vi "FPGAcode4.vi"() -> ()   [LabVIEW 2015]
uses:
  Limits_In.ctl
  Detector_Cluster.ctl
  <vilib>/Platform/TimedLoop/XDataNode/timing_clust.ctl
  <vilib>/Platform/TimedLoop/XDataNode/nitl_modes.ctl
  <vilib>/Platform/TimedLoop/XDataNode/wakeup.ctl
  Correlations.ctl
  <vilib>/rvi/Emulation/niFpgaSctlEmulationGetInTimedLoop.vi
  <vilib>/rvi/Emulation/niFpgaEmulationReportErrorSimple.vi
  <vilib>/rvi/Emulation/niFpgaGetClockAttributes.vi
  <vilib>/rvi/Emulation/niFpgaCriticalErrorInLSC.vi
  <vilib>/rvi/eio/common/nirviEmuTemplateMethod_errors.vi
  <vilib>/rvi/Emulation/niFpgaEmulationIsFPGAContextNoSignature.vi
  <vilib>/rvi/DataTransferAndStorage/Container/Common/niFpgaContainerGetUniqueNameForEmu.vi
  <vilib>/rvi/eio/common/nirviEmuReportErrorAndStop.vi
  <vilib>/rvi/Emulation/niFpgaProcessEmulError.vi
  <vilib>/Platform/TimedLoop/XDataNode/XDataNode.xnode
  <vilib>/eio/EIONode/EIONode.xnode
  <vilib>/rvi/DataTransferAndStorage/Container/XNode/niFpgaContainer.xnode
  <vilib>/rvi/DataTransferAndStorage/Handshake/Emulation/niFpgaHandshakeEmulation.vi
  <vilib>/Platform/TimedLoop/XDataNode/XDNodeRunTimeDep.lvlib
panel:
  in  "Charge Error Factor":fxp<+/-,11,1>=0.2001953125 format="%#.3g"
  in  "Calibrate":bool=TRUE
  in  "Limits":T1={"High Charge Limit"=4.54747350780585e-13, "Low Charge Limit"=0.0, "High Velocity Limit"=262143.0, "Low Velocity Limit"=0.0, "High Mass Limit"=7.27595761248936e-12, "Low Mass Limit"=0.0, "High Voltage"=2200000.0}
  in  "One Shot":bool
  in  "Threshold Factor":fxp<+,12,2>=1.150390625 format="%#.3g"
  in  "Armed":bool
  in  "User Trigger Distance":fxp<+/-,28,18> format="%#.3g"
  in  "User Trigger?":bool
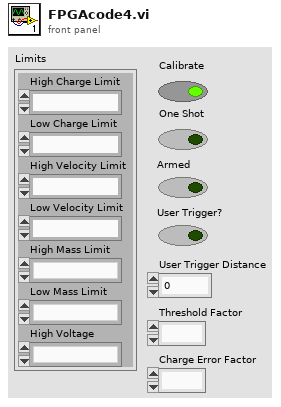
[diagram p1: front panel]
types:
  T1 = typedef "Limits_In.ctl" = cluster{"High Charge Limit":fxp<+,32,-41>, "Low Charge Limit":fxp<+,32,-41>, "High Velocity Limit":fxp<+,18,18>, "Low Velocity Limit":fxp<+,18,18>, "High Mass Limit":fxp<+,32,-37>, "Low Mass Limit":fxp<+,32,-37>, "High Voltage":fxp<+,22,22>}
  T2 = cluster{"[0]":fxp<+,16,1>, "[1]":fxp<+,16,1>, "[2]":fxp<+,16,1>, "[3]":fxp<+,16,1>, "[4]":fxp<+,16,1>, "[5]":fxp<+,16,1>, "[6]":fxp<+,16,1>, "[7]":fxp<+,16,1>, "[8]":fxp<+,16,1>, "[9]":fxp<+,16,1>, "[10]":fxp<+,16,1>}
  T3 = cluster{"[0]":i32, "[1]":i32, "[2]":i32, "[3]":i32, "[4]":i32, "[5]":i32, "[6]":i32, "[7]":i32, "[8]":i32, "[9]":i32, "[10]":i32}
  T4 = cluster{"[0]":cluster{"Detector Max Speed Count":i32, "Detector Min Speed Count":i32, "Gap Max Speed Count":i32, "Gap Min Speed Count":i32}, "[1]":cluster{"Detector Max Speed Count":i32, "Detector Min Speed Count":i32, "Gap Max Speed Count":i32, "Gap Min Speed Count":i32}, "[2]":cluster{"Detector Max Speed Count":i32, "Detector Min Speed Count":i32, "Gap Max Speed Count":i32, "Gap Min Speed Count":i32}, "[3]":cluster{"Detector Max Speed Count":i32, "Detector Min Speed Count":i32, "Gap Max Speed Count":i32, "Gap Min Speed Count":i32}, "[4]":cluster{"Detector Max Speed Count":i32, "Detector Min Speed Count":i32, "Gap Max Speed Count":i32, "Gap Min Speed Count":i32}, "[5]":cluster{"Detector Max Speed Count":i32, "Detector Min Speed Count":i32, "Gap Max Speed Count":i32, "Gap Min Speed Count":i32}, "[6]":cluster{"Detector Max Speed Count":i32, "Detector Min Speed Count":i32, "Gap Max Speed Count":i32, "Gap Min Speed Count":i32}, "[7]":cluster{"Detector Max Speed Count":i32, "Detector Min Speed Count":i32, "Gap Max Speed Count":i32, "Gap Min Speed Count":i32}, "[8]":cluster{"Detector Max Speed Count":i32, "Detector Min Speed Count":i32, "Gap Max Speed Count":i32, "Gap Min Speed Count":i32}, "[9]":cluster{"Detector Max Speed Count":i32, "Detector Min Speed Count":i32, "Gap Max Speed Count":i32, "Gap Min Speed Count":i32}, "[10]":cluster{"Detector Max Speed Count":i32, "Detector Min Speed Count":i32, "Gap Max Speed Count":i32, "Gap Min Speed Count":i32}}
  T5 = cluster{cluster{"[0]":i32, "[1]":i32, "[2]":i32, "[3]":i32, "[4]":i32, "[5]":i32, "[6]":i32, "[7]":i32, "[8]":i32, "[9]":i32, "[10]":i32}, cluster{"[0]":i32, "[1]":i32, "[2]":i32, "[3]":i32, "[4]":i32, "[5]":i32, "[6]":i32, "[7]":i32, "[8]":i32, "[9]":i32, "[10]":i32}, cluster{"[0]":i32, "[1]":i32, "[2]":i32, "[3]":i32, "[4]":i32, "[5]":i32, "[6]":i32, "[7]":i32, "[8]":i32, "[9]":i32, "[10]":i32}, cluster{"[0]":i32, "[1]":i32, "[2]":i32, "[3]":i32, "[4]":i32, "[5]":i32, "[6]":i32, "[7]":i32, "[8]":i32, "[9]":i32, "[10]":i32}}
  T6 = cluster{"Distance to PSU":fxp<+/-,64,37>, "Distance to end of PSU":fxp<+/-,64,37>, "Distance to DCS 2":fxp<+/-,64,37>, "Distance to DCS 1":fxp<+/-,64,37>, "Distance to front of LEIL Chamber":fxp<+/-,64,37>}
  T7 = typedef "Detector_Cluster.ctl" = cluster{"Det 1":i32, "Det 2":i32}
  T8 = cluster{"Filter 1":T7, "Filter 2":T7, "Filter 3":T7, "Filter 4":T7}
  T9 = cluster{"Detector Max Speed Count":i32, "Detector Min Speed Count":i32, "Gap Max Speed Count":i32, "Gap Min Speed Count":i32}[]
  T10 = cluster{"Filter 1":T7, "Filter 2":T7, "Filter 3":T7, "Filter 4":T7}[]
  T11 = typedef "XDNodeRunTimeDep.lvlib/timing_clust.ctl" = cluster{"Expected End [f-1]":u64, "Actual End [f-1]":u64, "Finished Late? [f-1]":bool, "Expected End [i-1]":u64, "Actual End [i-1]":u64, "Finished Late? [i-1]":bool, "Expected Start [i]":u64, "Actual Start [i]":u64, "Expected Start [f]":u64, "Actual Start [f]":u64, "Source Name":string, "Structure Name":string, "Period":i64, "Deadline":i64, "Offset":i64, "Start":i64, "Priority":i32, "Timeout":i32, "Mode":T12, "Wakeup Reason":T13, "Error":errorcluster, "Source Type":string, "Secondary Source Type":string, "Global End Time":u64, "Global Start Time":u64, "Frame Duration":u64, "Iteration Duration":u64, "Assigned CPU":i32, "I/O Scan Engine Mode":u32}
  T12 = typedef "XDNodeRunTimeDep.lvlib/nitl_modes.ctl" = enum32{"No Change", "Process missed periods, maintain original phase", "Discard missed periods, maintain original phase", "Process missed periods, ignore original phase", "Discard missed periods, ignore original phase"}
  T13 = typedef "XDNodeRunTimeDep.lvlib/wakeup.ctl" = enum32{"Normal", "Aborted", "Asynchronous wakeup", "Timing source error", "Timed loop error", "Timeout"}
  T14 = cluster{"IO Module\\AI 0":i16, "IO Module\\AI 1":i16}
  T15 = cluster{"First Detector Count":i32, "Detector Gap Count":i32, "Second Detector Count":i32, "Second Detector Final Count":i32}
  T16 = typedef "Correlations.ctl" = cluster{"First Correlation":i32, "Latest Correlation":i32}
  T17 = cluster{"Data":fxp<+/-,40,32>, "Data":fxp<+/-,40,32>}
  T18 = cluster{cluster{"Data":i16, "Data":i16}, cluster{"Det 1":i16, "Det 2":i16}, cluster{"Det 1":i16, "Det 2":i16}, cluster{"Det 1":i16, "Det 2":i16}}
  T19 = cluster{cluster{"Det 1":i16, "Det 2":i16}, cluster{"Det 1":i16, "Det 2":i16}, cluster{"Det 1":i16, "Det 2":i16}, cluster{"Det 1":i16, "Det 2":i16}}
  T20 = cluster{"Distance to PSU":fxp<+/-,64,69>, "Distance to end of PSU":fxp<+/-,64,69>, "Distance to DCS 2":fxp<+/-,64,69>, "Distance to DCS 1":fxp<+/-,64,69>, "Distance to front of LEIL Chamber":fxp<+/-,64,69>}
  T21 = cluster{"Distance to PSU":i32, "Distance to end of PSU":i32, "Distance to DCS 2":i32, "Distance to DCS 1":i32, "Distance to front of LEIL Chamber":i32}
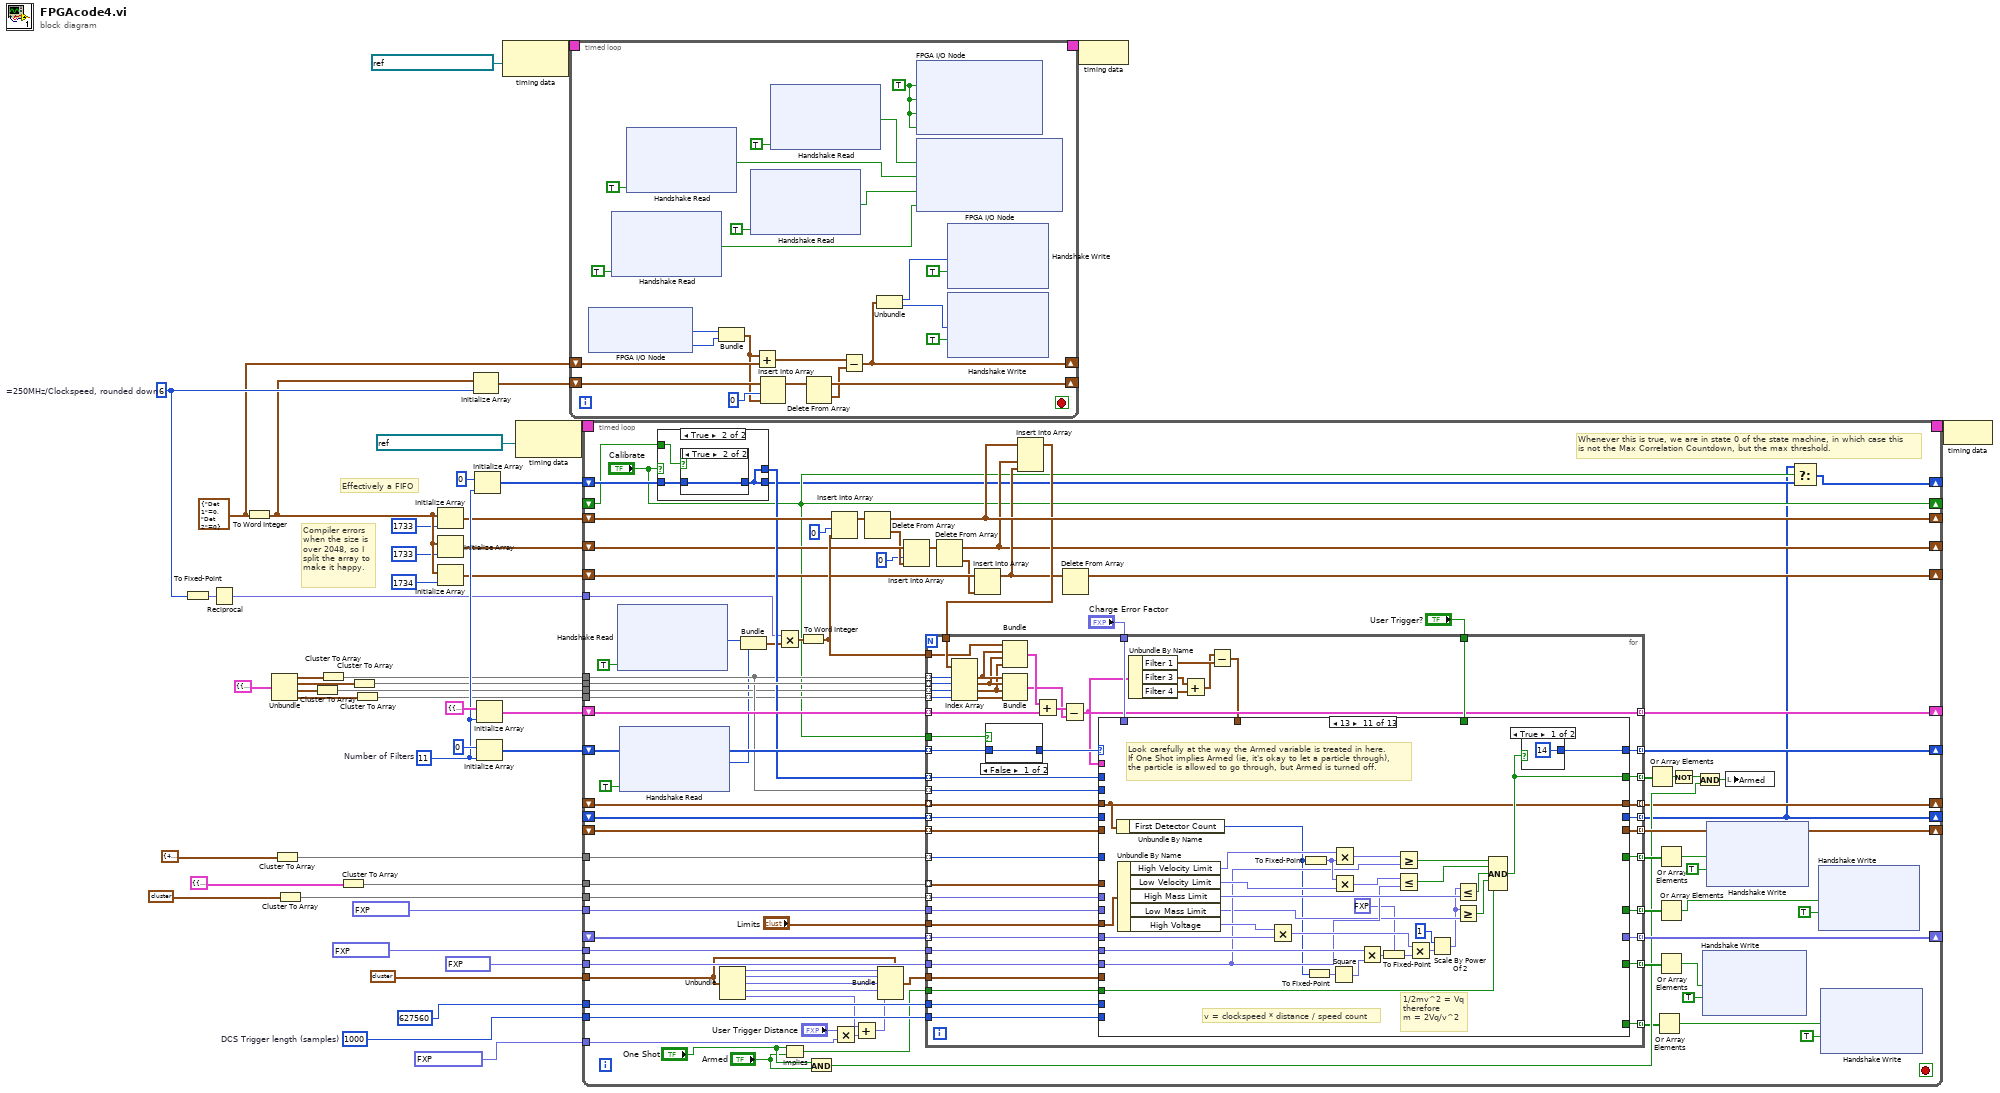
[diagram p0: block diagram]
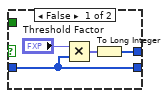
[diagram p2: hidden frame]
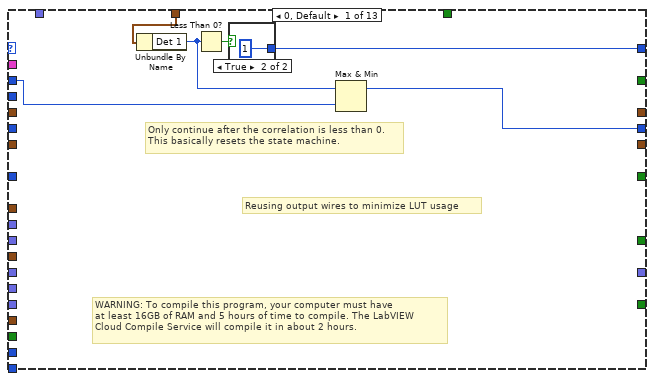
[diagram p5: hidden frame]
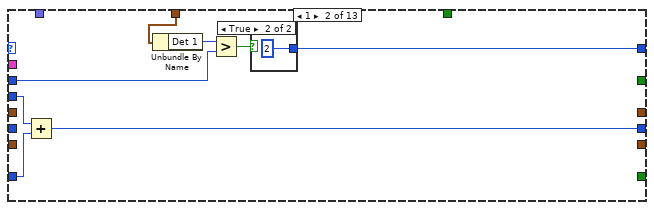
[diagram p7: hidden frame]
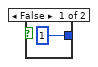
[diagram p8: hidden frame]
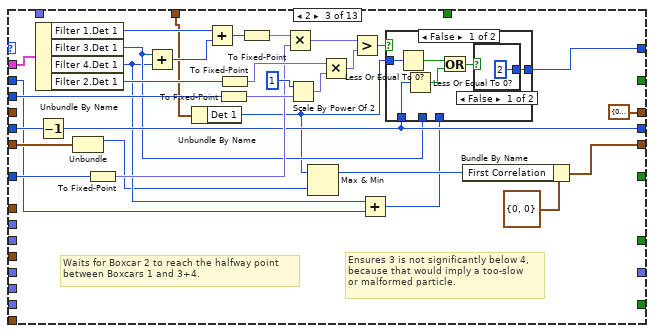
[diagram p9: hidden frame]
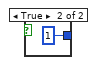
[diagram p10: hidden frame]
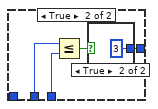
[diagram p11: hidden frame]
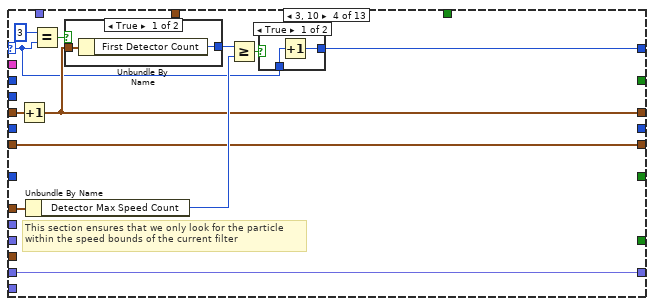
[diagram p13: hidden frame]
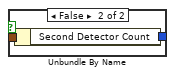
[diagram p14: hidden frame]
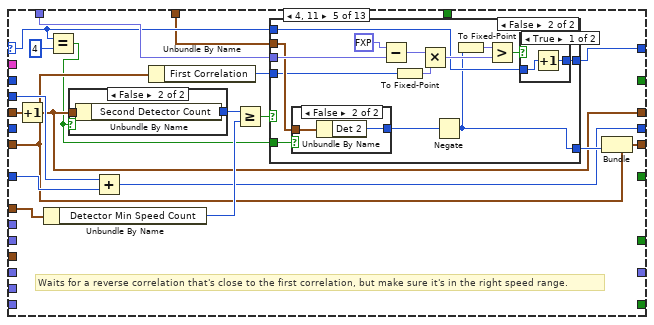
[diagram p16: hidden frame]
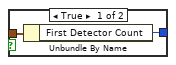
[diagram p17: hidden frame]
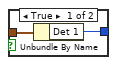
[diagram p19: hidden frame]
diagram:
  w39 = u8 6  # =250MHz/Clockspeed, rounded down
  w10 = u16 1000  # DCS Trigger length (samples)
  w7 = T7 {"Det 1"=0, "Det 2"=0} ("Detectors")
  w44 = 11  # Number of Filters
  # "Compiler errors\nwhen the size is\nover 2048, so I\nsplit the array to\nmake it happy."
  # "Effectively a FIFO"
  n1 = To Fixed-Point(number=w39) -> (fixed-point=w41:fxp<+,8,8>)  [unwired: 1 in]
  n2 = Reciprocal(x=w41) -> (1/x=w25:fxp<+,9,1>)
  n3 = To Word Integer(number=w7) -> (16bit integer=w6:cluster{"Det 1":i16, "Det 2":i16})
  n4 = Unbundle(T5 {{"[0]"=1200, "[1]"=1200, "[2]"=1200, "[3]"=1200, "[4]"=1200, "[5]"=650, "[6]"=306, "[7]"=140, "[8]"=62, "[9]"=26, "[10]"=10}, {"[0]"=5200, "[1]"=3559, "[2]"=2591, "[3]"=2020, "[4]"=1684, "[5]"=935, "[6]"=474, "[7]"=240, "[8]"=122, "[9]"=62, "[10]"=30}, {"[0]"=5800, "[1]"=4159, "[2]"=3191, "[3]"=2620, "[4]"=2284, "[5]"=1260, "[6]"=627, "[7]"=310, "[8]"=153, "[9]"=75, "[10]"=35}, {"[0]"=6400, "[1]"=4759, "[2]"=3791, "[3]"=3220, "[4]"=2884, "[5]"=1585, "[6]"=780, "[7]"=380, "[8]"=184, "[9]"=88, "[10]"=40}} ("output cluster")) -> (w37:T3, w36:T3, w35:T3, w34:T3)
  n5 = Cluster To Array(cluster=T3 {"[0]"=4000, "[1]"=2359, "[2]"=1391, "[3]"=820, "[4]"=484, "[5]"=285, "[6]"=168, "[7]"=99, "[8]"=59, "[9]"=35, "[10]"=20}) -> (array=w18:i32[])
  n6 = Cluster To Array(cluster=T2 {"[0]"=0.000823974609375, "[1]"=0.000823974609375, "[2]"=0.000823974609375, "[3]"=0.000823974609375, "[4]"=0.000823974609375, "[5]"=0.00152587890625, "[6]"=0.003265380859375, "[7]"=0.007080078125, "[8]"=0.015869140625, "[9]"=0.03704833984375, "[10]"=0.100006103515625} ("cluster 3")) -> (array=w16:fxp<+,16,1>[])
  n7 = Cluster To Array(cluster=w35) -> (array=w22:i32[])
  n8 = Cluster To Array(cluster=w37) -> (array=w24:i32[])
  n9 = Cluster To Array(cluster=T4 {"[0]"={"Detector Max Speed Count"=42000, "Detector Min Speed Count"=84000, "Gap Max Speed Count"=78000, "Gap Min Speed Count"=156000}, "[1]"={"Detector Max Speed Count"=21477, "Detector Min Speed Count"=42953, "Gap Max Speed Count"=39885, "Gap Min Speed Count"=79770}, "[2]"={"Detector Max Speed Count"=10982, "Detector Min Speed Count"=21964, "Gap Max Speed Count"=20395, "Gap Min Speed Count"=40790}, "[3]"={"Detector Max Speed Count"=5616, "Detector Min Speed Count"=11231, "Gap Max Speed Count"=10429, "Gap Min Speed Count"=20858}, "[4]"={"Detector Max Speed Count"=2872, "Detector Min Speed Count"=5743, "Gap Max Speed Count"=5333, "Gap Min Speed Count"=10666}, "[5]"={"Detector Max Speed Count"=1468, "Detector Min Speed Count"=2937, "Gap Max Speed Count"=2727, "Gap Min Speed Count"=5454}, "[6]"={"Detector Max Speed Count"=751, "Detector Min Speed Count"=1502, "Gap Max Speed Count"=1394, "Gap Min Speed Count"=2789}, "[7]"={"Detector Max Speed Count"=384, "Detector Min Speed Count"=768, "Gap Max Speed Count"=713, "Gap Min Speed Count"=1426}, "[8]"={"Detector Max Speed Count"=196, "Detector Min Speed Count"=393, "Gap Max Speed Count"=365, "Gap Min Speed Count"=729}, "[9]"={"Detector Max Speed Count"=100, "Detector Min Speed Count"=201, "Gap Max Speed Count"=186, "Gap Min Speed Count"=373}, "[10]"={"Detector Max Speed Count"=51, "Detector Min Speed Count"=103, "Gap Max Speed Count"=95, "Gap Min Speed Count"=191}} ("cluster 2")) -> (array=w17:T9)
  n10 = Cluster To Array(cluster=w36) -> (array=w23:i32[])
  n11 = Cluster To Array(cluster=w34) -> (array=w21:i32[])
  n12 = Initialize Array(w6, 1733 ("dimension size")) -> (w26:cluster{"Det 1":i16, "Det 2":i16}[])
  n13 = Initialize Array(w6, 1733 ("dimension size")) -> (w5:cluster{"Det 1":i16, "Det 2":i16}[])
  n14 = Initialize Array(w6, 1734 ("dimension size")) -> (w4:cluster{"Det 1":i16, "Det 2":i16}[])
  n15 = Initialize Array(w6, w39) -> (w40:cluster{"Det 1":i16, "Det 2":i16}[])
  n16 = Initialize Array(0 ("Thresholds in"), w44) -> (w27:i32[])
  n17 = Initialize Array(T8 {"Filter 1"={"Det 1"=0, "Det 2"=0}, "Filter 2"={"Det 1"=0, "Det 2"=0}, "Filter 3"={"Det 1"=0, "Det 2"=0}, "Filter 4"={"Det 1"=0, "Det 2"=0}} ("cluster"), w44) -> (w20:T10)
  n18 = Initialize Array(u8 0, w44) -> (w19:u8[])
  n19 = node-c288(refnum<k21> "IO Module\\Data Clock" ("Source Name")) -> (w43:T11)
  n20 = node-c288(refnum<k21> "40 MHz Onboard Clock" ("Source Name")) -> (w29:T11)
  n21 = timed-loop {
    timing: w43 -> [_]
    timing-out: [_] -> w42
    shift-right: [w61] -> _
    shift-left: w7 -> [w70]
    shift-right: [w63] -> _
    shift-left: w40 -> [w68]
    stop <- _ stop-if-true
    w48 = TRUE ("IO Module\\PFI Enable")
    n22 = xnode "FPGA I/O Node"() -> ("IO Module\\AI 0"=w67:i16, "IO Module\\AI 1"=w66:i16)  [unwired: 2 in, 2 out]
    n23 = xnode ("Handshake Read")("Ready for Output"=TRUE) -> ("Data"=w56:bool)  [unwired: 1 in, 2 out]
    n24 = xnode ("Handshake Read")("Ready for Output"=TRUE) -> ("Data"=w52:bool)  [unwired: 1 in, 2 out]
    n25 = Bundle("IO Module\\AI 0"=w67, "IO Module\\AI 1"=w66) -> (w65:T14)  [unwired: 1 in]
    n26 = xnode ("Handshake Read")("Ready for Output"=TRUE) -> ("Data"=w55:bool)  [unwired: 1 in, 2 out]
    n27 = Add(x=w65, y=w70) -> (x+y=w69:T7)
    n28 = Insert Into Array(array=w68, index=0, new element=w65) -> (w64:cluster{"Det 1":i16, "Det 2":i16}[])
    n29 = xnode ("Handshake Read")("Ready for Output"=TRUE) -> ("Data"=w49:bool)  [unwired: 1 in, 2 out]
    n30 = Delete From Array(array=w64) -> (deleted portion=w62:cluster{"Det 1":i16, "Det 2":i16}, array with subset deleted=w63:cluster{"Det 1":i16, "Det 2":i16}[])  [unwired: 2 in]
    n31 = Subtract(x=w69, y=w62) -> (x-y=w61:T7)
    n32 = Unbundle(w61) -> ("Det 1"=w59:i32, "Det 2"=w57:i32)
    n33 = xnode "FPGA I/O Node"("IO Module\\PFI 0 WE"=w48, "IO Module\\PFI 1 WE"=w48, "IO Module\\PFI 2 WE"=w48, "IO Module\\PFI 3 WE"=w48) -> ()  [unwired: 4 in, 4 out]
    n34 = xnode "FPGA I/O Node"("IO Module\\PFI 0 Wr Data"=w49, "IO Module\\PFI 1 Wr Data"=w52, "IO Module\\PFI 2 Wr Data"=w55, "IO Module\\PFI 3 Wr Data"=w56) -> ()  [unwired: 4 in, 4 out]
    n35 = xnode ("Handshake Write")("Data"=w59, "Input Valid"=TRUE) -> ()  [unwired: 1 in, 2 out]
    n36 = xnode ("Handshake Write")("Data"=w57, "Input Valid"=TRUE) -> ()  [unwired: 1 in, 2 out]
  }
  n37 = timed-loop {
    shift-right: [w83] -> _
    shift-left: w26 -> [w159]
    shift-right: [w112] -> _
    shift-left: w20 -> [w156]
    shift-right: [w107] -> _
    shift-left: w19 -> [w158]
    shift-right: [w113] -> _
    shift-left: _ -> [w157]
    tunnel: w17 -> [w155]
    shift-right: [w154] -> _
    shift-left: _ -> [w153]
    tunnel: w24 -> [w111]
    tunnel: w23 -> [w152]
    tunnel: w18 -> [w151]
    tunnel: w16 -> [w150]
    shift-right: [w149] -> _
    shift-left: _ -> [w148]
    tunnel: fxp<+,32,-43> 9.525990075777386e-16 ("fixed-point 2") -> [w147]
    tunnel: fxp<+,32,-49> 2.2727300016438096e-16 ("fixed-point 3") -> [w146]
    tunnel: fxp<+,28,28> 32400000.0 ("fixed-point") -> [w145]
    tunnel: T6 {"Distance to PSU"=1.2345678955316544, "Distance to end of PSU"=2.4691357985138893, "Distance to DCS 2"=3.229876533150673, "Distance to DCS 1"=-1.677654318511486, "Distance to front of LEIL Chamber"=5.305777758359909} ("x/y") -> [w139]
    shift-right: [w74] -> _
    shift-left: w27 -> [w144]
    shift-right: ["Calibrate"] -> _
    shift-left: _ -> [w143]
    tunnel: w10 -> [w142]
    tunnel: 627560 ("32bit integer") -> [w141]
    tunnel: fxp<+,32,1> 1.2345679011195898 ("1/x") -> [w140]
    shift-right: [w75] -> _
    shift-left: _ -> [w110]
    tunnel: w21 -> [w109]
    tunnel: w22 -> [w108]
    timing: w29 -> [_]
    timing-out: [_] -> w28
    tunnel: w25 -> [w105]
    shift-right: [w78] -> _
    shift-left: w5 -> [w89]
    shift-right: [w79] -> _
    shift-left: w4 -> [w88]
    stop <- _ stop-if-true
    # "Whenever this is true, we are in state 0 of the state machine, in which case this\nis not the Max Correlation Countdown, but the max threshold."
    n38 = xnode ("Handshake Read")("Ready for Output"=TRUE) -> ("Data"=w93:i32)  [unwired: 1 in, 2 out]
    n39 = xnode ("Handshake Read")("Ready for Output"=TRUE) -> ("Data"=w92:i32)  [unwired: 1 in, 2 out]
    n40 = case shown="True" "Calibrate" {
      tunnel: w144 -> [w161 w165]
      tunnel: [w161 w164] -> w76
      tunnel: w143 -> [_ w166]
      tunnel: [w160 w164] -> w114
      frame False {
        n41 = Multiply(x="Threshold Factor", y=w161) -> (x*y=w162:fxp<+/-,44,34>[])
        n42 = To Long Integer(number=w162) -> (32bit integer=w160:i32[])
      }
      frame True {
        n43 = case shown="True" w166 {
          tunnel: w165 -> [_ w167]
          tunnel: [_ w167] -> w164
          frame False {
          }
          frame True {
          }
        }
      }
    }
    n44 = Unbundle(w139) -> ("Distance to PSU"=w133:fxp<+/-,64,37>, "Distance to end of PSU"=w132:fxp<+/-,64,37>, "Distance to DCS 2"=w131:fxp<+/-,64,37>, "Distance to DCS 1"=w128:fxp<+/-,64,37>, "Distance to front of LEIL Chamber"=w127:fxp<+/-,64,37>)
    n45 = Bundle("Data"=w93, "Data"=w92) -> (w91:cluster{"Data":i32, "Data":i32})  [unwired: 1 in]
    n46 = Multiply(x=w105, y=w91) -> (x*y=w106:T17)
    n47 = Implies(1:"Armed", 2:"One Shot") -> (0:w135:bool)
    n48 = To Word Integer(number=w106) -> (16bit integer=w104:cluster{"Data":i16, "Data":i16})
    n49 = And(x="One Shot", y="Armed") -> (x .and. y?=w119:bool)
    n50 = Insert Into Array(array=w159, index=0, new element=w104) -> (w82:cluster{"Det 1":i16, "Det 2":i16}[])
    n51 = Multiply(x="User Trigger Distance", y=w140) -> (x*y=w129:fxp<+/-,60,19>)
    n52 = Add(x=w127, y=w129) -> (x+y=w126:fxp<+/-,64,38>)
    n53 = Delete From Array(array=w82) -> (deleted portion=w87:cluster{"Det 1":i16, "Det 2":i16}, array with subset deleted=w83:cluster{"Det 1":i16, "Det 2":i16}[])  [unwired: 2 in]
    n54 = Bundle(cluster=w139, "Distance to PSU"=w133, "Distance to end of PSU"=w132, "Distance to DCS 2"=w131, "Distance to DCS 1"=w128, "Distance to front of LEIL Chamber"=w126) -> (w130:T6)
    n55 = Insert Into Array(array=w89, index=0, new element=w87) -> (w86:cluster{"Det 1":i16, "Det 2":i16}[])
    n56 = Delete From Array(array=w86) -> (deleted portion=w85:cluster{"Det 1":i16, "Det 2":i16}, array with subset deleted=w78:cluster{"Det 1":i16, "Det 2":i16}[])  [unwired: 2 in]
    n57 = Insert Into Array(array=w88, new element=w85) -> (w80:cluster{"Det 1":i16, "Det 2":i16}[])  [unwired: 1 in]
    n58 = Insert Into Array(array=w83, new element #1=w78, new element #2=w80) -> (w81:cluster{"Det 1":i16, "Det 2":i16}[])  [unwired: 1 in]
    n59 = for {
      tunnel: w81 -> [w219]
      tunnel: [w169] -> w112 mode=indexing
      tunnel: w158 -> [w175] mode=indexing
      tunnel: [w218] -> w107 mode=indexing
      tunnel: w114 -> [w181] mode=indexing
      tunnel: [w217] -> w113 mode=indexing
      tunnel: w157 -> [w216] mode=indexing
      tunnel: w156 -> [w210] mode=indexing
      tunnel: w104 -> [w215]
      tunnel: w155 -> [w206] mode=indexing
      tunnel: [w205] -> w154 mode=indexing
      tunnel: w153 -> [w204] mode=indexing
      tunnel: w111 -> [w203] mode=indexing
      tunnel: w152 -> [w179] mode=indexing
      tunnel: w108 -> [w202] mode=indexing
      tunnel: w109 -> [w201] mode=indexing
      tunnel: w111 -> [w183] mode=indexing
      tunnel: w151 -> [w182] mode=indexing
      tunnel: "Charge Error Factor" -> [w200]
      tunnel: w150 -> [w199] mode=indexing
      tunnel: "Limits" -> [w198]
      tunnel: [w197] -> w149 mode=indexing
      tunnel: w148 -> [w196] mode=indexing
      tunnel: w147 -> [w195]
      tunnel: w146 -> [w194]
      tunnel: w145 -> [w193]
      tunnel: w130 -> [w192]
      tunnel: w135 -> [w191]
      tunnel: w142 -> [w189]
      tunnel: w141 -> [w190]
      tunnel: [w188] -> w125 mode=indexing
      tunnel: [w187] -> w124 mode=indexing
      tunnel: [w186] -> w123 mode=indexing
      tunnel: [w185] -> w122 mode=indexing
      tunnel: "User Trigger?" -> [w184]
      tunnel: "Calibrate" -> [w176]
      tunnel: [w180] -> w75 mode=indexing
      tunnel: w110 -> [w178] mode=indexing
      tunnel: [w177] -> w90 mode=indexing
      n60 = Index Array(array=w219, index #1=w203, index #2=w179, index #3=w202, index #4=w201) -> (element #1=w213:cluster{"Det 1":i16, "Det 2":i16}, element #2=w212:cluster{"Det 1":i16, "Det 2":i16}, element #3=w211:cluster{"Det 1":i16, "Det 2":i16}, element #4=w214:cluster{"Det 1":i16, "Det 2":i16})
      n61 = case shown="False" w176 {
        tunnel: w175 -> [w220 _]
        tunnel: [w220 _] -> w174
        frame False {
        }
        frame True {
        }
      }
      n62 = Bundle(w215, w213, w212, w211) -> (w209:T18)  [unwired: 1 in]
      n63 = Bundle(w213, w212, w211, w214) -> (w207:T19)  [unwired: 1 in]
      n64 = Add(x=w209, y=w210) -> (x+y=w208:T8)
      n65 = Subtract(x=w208, y=w207) -> (x-y=w169:T8)
      n66 = Unbundle By Name(w169) -> ("Filter 1"=w173:T7, "Filter 3"=w172:T7, "Filter 4"=w171:T7)
      n67 = Add(x=w172, y=w171) -> (x+y=w170:T7)
      n68 = Subtract(x=w170, y=w173) -> (x-y=w168:T7)
      n69 = case shown="13" w174 {
        selector: w174 -> [_ _ _ w283 w304 w348 _ _ _ _ _ _ _]
        tunnel: w181 -> [w225 w235 w243 _ _ _ _ _ _ _ _ _ _]
        tunnel: [w226 w234 w267 w289 w313 w389 w431 w445 w460 w519 w546 u8 15 ("Det 3") w610] -> w218
        tunnel: w183 -> [_ w233 w261 _ w315 w381 _ _ w462 w511 _ w578 _]
        tunnel: [_ _ T15 {"First Detector Count"=0, "Detector Gap Count"=0, "Second Detector Count"=0, "Second Detector Final Count"=0} ("Cutoffs") w286 w305 w353 w421 w442 w454 w484 w529 w569 w608] -> w217
        tunnel: w216 -> [_ _ _ w287 w310 w358 w422 w443 w457 w490 w529 w568 w609]
        tunnel: w178 -> [_ _ w268 _ _ w390 _ _ _ w520 _ _ w591]
        tunnel: w169 -> [_ _ w254 _ _ w374 _ _ _ w505 _ _ _]
        tunnel: w206 -> [_ _ _ w293 w319 w359 _ w449 w466 w489 _ _ _]
        tunnel: w204 -> [_ _ w246 w288 w307 w357 w424 w444 w456 w498 _ _ _]
        tunnel: w182 -> [_ w232 w262 _ w314 w382 _ _ w461 w512 _ w572 _]
        tunnel: w200 -> [_ _ _ _ w316 w367 _ _ w463 w499 _ _ _]
        tunnel: w199 -> [_ _ _ _ _ _ w436 _ _ _ _ _ _]
        tunnel: w198 -> [_ _ _ _ _ _ w439 _ _ _ w557 _ _]
        tunnel: [_ _ _ w285 _ _ w419 w441 w453 w482 _ _ _] -> w197
        tunnel: w196 -> [_ _ _ w285 _ _ _ w441 w453 w482 w535 _ _]
        tunnel: w195 -> [_ _ _ _ _ _ _ _ _ _ w556 _ _]
        tunnel: w194 -> [_ _ _ _ _ _ w429 _ _ _ _ _ _]
        tunnel: w193 -> [_ _ _ _ _ _ _ _ _ _ w534 _ _]
        tunnel: w192 -> [_ _ _ _ _ _ _ _ _ _ _ w581 _]
        tunnel: w191 -> [_ _ _ _ _ _ _ _ _ _ w540 _ _]
        tunnel: w190 -> [_ _ _ _ _ _ _ _ _ _ _ w575 _]
        tunnel: w189 -> [_ _ _ _ _ _ _ _ _ _ _ _ w588]
        tunnel: [_ _ _ _ _ _ _ _ _ _ _ _ w607] -> w188
        tunnel: [_ _ _ _ _ _ _ _ _ _ _ _ w606] -> w187
        tunnel: [_ _ _ _ _ _ _ _ _ _ _ _ w590] -> w186
        tunnel: [_ _ _ _ _ _ _ _ _ _ w539 _ _] -> w185
        tunnel: w184 -> [_ _ _ _ _ _ _ _ _ _ _ _ w592]
        tunnel: [w224 w231 w250 _ w306 w370 _ _ w455 w501 _ _ w584] -> w180
        tunnel: [_ _ w256 w288 w309 w376 w423 w444 w456 w498 _ _ _] -> w205
        tunnel: [_ _ _ _ _ _ _ _ _ _ _ _ w589] -> w177
        tunnel: w168 -> [w222 w229 w238 _ w301 w346 _ _ w452 w481 _ _ _]
        frame 0, Default {
          # "Reusing output wires to minimize LUT usage"
          # "WARNING: To compile this program, your computer must have\nat least 16GB of RAM and 5 hours of time to compile. The LabVIEW\nCloud Compile Service will compile it in about 2 hours."
          # "Only continue after the correlation is less than 0.\nThis basically resets the state machine."
          n70 = Unbundle By Name(w222) -> ("Det 1"=w221:i32)
          n71 = Less Than 0?(x=w221) -> (x < 0?=w223:bool)
          n72 = case shown="True" w223 {
            tunnel: [_ u8 1 ("Det 3")] -> w226
            frame False {
            }
            frame True {
            }
          }
          n73 = Max & Min(x=w221, y=w225) -> (max(x,y)=w224:i32)  [unwired: 1 out]
        }
        frame 1 {
          n74 = Add(x=w233, y=w232) -> (x+y=w231:i32)
          n75 = Unbundle By Name(w229) -> ("Det 1"=w228:i32)
          n76 = Greater?(x=w228, y=w235) -> (0:w230:bool)
          n77 = case shown="True" w230 {
            tunnel: [u8 1 ("Det 3") u8 2 ("Det 3")] -> w234
            frame False {
            }
            frame True {
            }
          }
        }
        frame 2 {
          # "Ensures 3 is not significantly below 4,\nbecause that would imply a too-slow\nor malformed particle."
          # "Waits for Boxcar 2 to reach the halfway point\nbetween Boxcars 1 and 3+4."
          n78 = Unbundle By Name(w254) -> ("Filter 1.Det 1"=w264:i32, "Filter 3.Det 1"=w242:i32, "Filter 4.Det 1"=w241:i32, "Filter 2.Det 1"=w258:i32)
          n79 = Decrement(x=w268) -> (x-1=w250:i32)
          n80 = Unbundle(w246) -> ("First Correlation"=w240:i32)  [unwired: 1 out]
          n81 = To Fixed-Point(number=w262) -> (fixed-point=w251:fxp<+/-,32,32>)  [unwired: 1 in]
          n82 = Add(x=w242, y=w241) -> (x+y=w265:i32)
          n83 = Unbundle By Name(w238) -> ("Det 1"=w239:i32)
          n84 = Add(x=w264, y=w265) -> (x+y=w266:i32)
          n85 = To Fixed-Point(number=w261) -> (fixed-point=w252:fxp<+/-,32,32>)  [unwired: 1 in]
          n86 = To Fixed-Point(number=w258) -> (fixed-point=w253:fxp<+/-,32,32>)  [unwired: 1 in]
          n87 = To Fixed-Point(number=w266) -> (fixed-point=w255:fxp<+/-,32,32>)  [unwired: 1 in]
          n88 = Multiply(x=w255, y=w251) -> (x*y=w263:fxp<+/-,64,64>)
          n89 = Scale By Power Of 2(n=i16 1, x=w252) -> (x*2^n=w259:fxp<+/-,32,32>)
          n90 = Max & Min(x=w239, y=w240) -> (max(x,y)=w247:i32)  [unwired: 1 out]
          n91 = Multiply(x=w253, y=w259) -> (x*y=w257:fxp<+/-,64,64>)
          n92 = Greater?(x=w263, y=w257) -> (0:w248:bool)
          n93 = Add(x=w241, y=w243) -> (x+y=w244:i32)
          n94 = case shown="False" w248 {
            tunnel: [w274 w280] -> w267
            tunnel: w250 -> [w270 _]
            tunnel: w239 -> [w269 _]
            tunnel: w244 -> [_ w278]
            tunnel: w242 -> [_ w279]
            frame False {
              n95 = Less Or Equal To 0?(x=w269) -> (x <= 0?=w272:bool)
              n96 = Less Or Equal To 0?(x=w270) -> (x <= 0?=w271:bool)
              n97 = Or(x=w272, y=w271) -> (x .or. y?=w273:bool)
              n98 = case shown="False" w273 {
                tunnel: [u8 2 ("Det 3") u8 1 ("Det 3")] -> w274
                frame False {
                }
                frame True {
                }
              }
            }
            frame True {
              n99 = Less Or Equal?(x=w279, y=w278) -> (x <= y?=w277:bool)
              n100 = case shown="True" w277 {
                tunnel: [_ u8 3 ("Det 3")] -> w280
                frame False {
                }
                frame True {
                }
              }
            }
          }
          n101 = Bundle By Name(cluster=T16 {"First Correlation"=0, "Latest Correlation"=0}, "First Correlation"=w247) -> (w256:T16)
        }
        frame 3, 10 {
          # "This section ensures that we only look for the particle\nwithin the speed bounds of the current filter"
          n102 = Increment(x=w287) -> (x+1=w286:T15)
          n103 = Unbundle By Name(w293) -> ("Detector Max Speed Count"=w291:i32)
          n104 = Equal?(x=u8 3, y=w283) -> (x = y?=w284:bool)
          n105 = case shown="True" w284 {
            tunnel: [w295 w297] -> w292
            tunnel: w286 -> [w294 w296]
            frame True {
              n106 = Unbundle By Name(w294) -> ("First Detector Count"=w295:i32)
            }
            frame False {
              n107 = Unbundle By Name(w296) -> ("Second Detector Count"=w297:i32)
            }
          }
          n108 = Greater Or Equal?(x=w292, y=w291) -> (x >= y?=w290:bool)
          n109 = case shown="True" w290 {
            tunnel: [w299 w300] -> w289
            tunnel: w283 -> [w298 w300]
            frame True {
              n110 = Increment(x=w298) -> (x+1=w299:u8)
            }
            frame False {
            }
          }
        }
        frame 4, 11 {
          # "Waits for a reverse correlation that's close to the first correlation, but make sure it's in the right speed range."
          n111 = Increment(x=w310) -> (x+1=w305:T15)
          n112 = Unbundle By Name(w319) -> ("Detector Min Speed Count"=w318:i32)
          n113 = Equal?(x=w304, y=u8 4 ("x")) -> (x = y?=w302:bool)
          n114 = case shown="False" w302 {
            tunnel: [w321 w323] -> w311
            tunnel: w305 -> [w320 w322]
            frame True {
              n115 = Unbundle By Name(w320) -> ("First Detector Count"=w321:i32)
            }
            frame False {
              n116 = Unbundle By Name(w322) -> ("Second Detector Count"=w323:i32)
            }
          }
          n117 = Add(x=w315, y=w314) -> (x+y=w306:i32)
          n118 = Unbundle By Name(w307) -> ("First Correlation"=w312:i32)
          n119 = Greater Or Equal?(x=w311, y=w318) -> (x >= y?=w317:bool)
          n120 = case shown="False" w317 {
            tunnel: [_ w337] -> w313
            tunnel: w316 -> [_ w336]
            tunnel: w301 -> [_ w333]
            tunnel: w312 -> [_ w328]
            tunnel: [_ w324] -> w308
            tunnel: w304 -> [_ w327]
            tunnel: w302 -> [_ w326]
            frame True {
            }
            frame False {
              n121 = case shown="False" w326 {
                tunnel: w333 -> [w339 w341]
                tunnel: [w338 w340] -> w325
                frame True {
                  n122 = Unbundle By Name(w339) -> ("Det 1"=w338:i32)
                }
                frame False {
                  n123 = Unbundle By Name(w341) -> ("Det 2"=w340:i32)
                }
              }
              n124 = Subtract(x=fxp<+,1,1> 1.0, y=w336) -> (x-y=w334:fxp<+,12,2>)
              n125 = To Fixed-Point(number=w328) -> (fixed-point=w330:fxp<+/-,32,32>)  [unwired: 1 in]
              n126 = Multiply(x=w334, y=w330) -> (x*y=w332:fxp<+/-,43,33>)
              n127 = Negate(x=w325) -> (-x=w324:i32)
              n128 = To Fixed-Point(number=w324) -> (fixed-point=w329:fxp<+/-,32,32>)  [unwired: 1 in]
              n129 = Greater?(x=w329, y=w332) -> (0:w331:bool)
              n130 = case shown="True" w331 {
                tunnel: [w342 w343] -> w337
                tunnel: w327 -> [w342 w343]
                frame True {
                  n131 = Increment(x=w342) -> ()  [unwired: 1 out]
                }
                frame False {
                }
              }
            }
          }
          n132 = Bundle(cluster=w307, "Latest Correlation"=w308) -> (w309:T16)  [unwired: 1 in]
        }
        frame 5, 12 {
          # "This is used for two cases to save LUTs"
          # "Waits for Boxcar 2 to reach the halfway point\nbetween Boxcars 1 and 3+4."
          n133 = Equal?(x=u8 5, y=w348) -> (x = y?=w347:bool)
          n134 = case shown="False" w347 {
            tunnel: [w403 w408] -> w387
            tunnel: [w402 w407] -> w386
            tunnel: [w401 w406] -> w384
            tunnel: [w400 w405] -> w378
            tunnel: w374 -> [w399 w404]
            frame True {
              n135 = Unbundle By Name(w399) -> ("Filter 1.Det 1"=w401:i32, "Filter 3.Det 1"=w403:i32, "Filter 4.Det 1"=w402:i32, "Filter 2.Det 1"=w400:i32)
            }
            frame False {
              n136 = Unbundle By Name(w404) -> ("Filter 1.Det 2"=w406:i32, "Filter 3.Det 2"=w408:i32, "Filter 4.Det 2"=w407:i32, "Filter 2.Det 2"=w405:i32)
            }
          }
          n137 = case shown="True" w347 {
            tunnel: w358 -> [w394 w397]
            tunnel: [w393 w398] -> w356
            tunnel: w346 -> [w392 w396]
            tunnel: [w391 w395] -> w345
            frame True {
              n138 = Unbundle By Name(w394) -> ("First Detector Count"=w393:i32)
              n139 = Unbundle By Name(w392) -> ("Det 1"=w391:i32)
            }
            frame False {
              n140 = Unbundle By Name(w397) -> ("Second Detector Count"=w398:i32)
              n141 = Unbundle By Name(w396) -> ("Det 2"=w395:i32)
            }
          }
          n142 = Unbundle By Name(w359) -> ("Detector Min Speed Count"=w355:i32)
          n143 = Increment(x=w358) -> (x+1=w368:T15)
          n144 = To Fixed-Point(number=w382) -> (fixed-point=w371:fxp<+/-,32,32>)  [unwired: 1 in]
          n145 = Decrement(x=w390) -> (x-1=w370:i32)
          n146 = Increment(x=w367) -> (x+1=w364:fxp<+,11,1>)
          n147 = Add(x=w387, y=w386) -> (x+y=w385:i32)
          n148 = Unbundle(w357) -> ("First Correlation"=w366:i32, "Latest Correlation"=w351:i32)
          n149 = To Fixed-Point(number=w366) -> (fixed-point=w365:fxp<+/-,32,32>)  [unwired: 1 in]
          n150 = Add(x=w384, y=w385) -> (x+y=w388:i32)
          n151 = To Fixed-Point(number=w378) -> (fixed-point=w373:fxp<+/-,32,32>)  [unwired: 1 in]
          n152 = To Fixed-Point(number=w381) -> (fixed-point=w372:fxp<+/-,32,32>)  [unwired: 1 in]
          n153 = Multiply(x=w365, y=w364) -> (x*y=w362:fxp<+/-,43,33>)
          n154 = To Fixed-Point(number=w388) -> (fixed-point=w375:fxp<+/-,32,32>)  [unwired: 1 in]
          n155 = Negate(x=w345) -> (-x=w344:i32)
          n156 = Greater Or Equal?(x=w356, y=w355) -> (x >= y?=w354:bool)
          n157 = Multiply(x=w375, y=w371) -> (x*y=w383:fxp<+/-,64,64>)
          n158 = To Fixed-Point(number=w344) -> (fixed-point=w363:fxp<+/-,32,32>)  [unwired: 1 in]
          n159 = Scale By Power Of 2(n=i16 1, x=w372) -> (x*2^n=w379:fxp<+/-,32,32>)
          n160 = Greater?(x=w363, y=w362) -> (0:w361:bool)
          n161 = Max & Min(x=w344, y=w351) -> (max(x,y)=w350:i32)  [unwired: 1 out]
          n162 = Multiply(x=w373, y=w379) -> (x*y=w377:fxp<+/-,64,64>)
          n163 = Or(x=w361, y=w354) -> (x .or. y?=w360:bool)
          n164 = Less?(x=w383, y=w377) -> (x < y?=w369:bool)
          n165 = case shown="False" w369 {
            tunnel: [w414 w416] -> w389
            tunnel: w370 -> [w411 _]
            tunnel: w360 -> [w410 _]
            tunnel: w348 -> [w409 w417]
            frame False {
              n166 = Less Or Equal To 0?(x=w411) -> (x <= 0?=w412:bool)
              n167 = Or(x=w410, y=w412) -> (x .or. y?=w413:bool)
              n168 = case shown="False" w413 {
                tunnel: [w415 _] -> w414
                tunnel: w409 -> [w415 _]
                frame False {
                }
                frame True {
                }
              }
            }
            frame True {
              n169 = Increment(x=w417) -> (x+1=w416:u8)
            }
          }
          n170 = Bundle By Name(cluster=w357, "Latest Correlation"=w350) -> (w376:T16)
          n171 = Bundle By Name(cluster=w368, "Detector Gap Count"=0) -> (w353:T15)
        }
        frame 6 {
          # "q = ADC value / CSA sensitivity"
          # "Ensures the charge is good"
          n172 = Unbundle(w424) -> ("First Correlation"=w438:i32, "Latest Correlation"=w437:i32)
          n173 = Unbundle By Name(w439) -> ("High Charge Limit"=w418:fxp<+,32,-41>, "Low Charge Limit"=w435:fxp<+,32,-41>)
          n174 = Add(x=w438, y=w437) -> (x+y=w427:i32)
          n175 = Increment(x=w422) -> (x+1=w421:T15)
          n176 = Scale By Power Of 2(n=i16 -1, x=w427) -> (x*2^n=w425:i32)
          n177 = To Fixed-Point(number=w425) -> (fixed-point=w426:fxp<+/-,32,32>)  [unwired: 1 in]
          n178 = Multiply(x=w426, y=w436) -> (x*y=w430:fxp<+/-,47,32>)
          n179 = Multiply(x=w430, y=w429) -> (x*y=w420:fxp<+/-,64,-17>)
          n180 = Bundle(cluster=w424, "First Correlation"=w425) -> (w423:T16)  [unwired: 1 in]
          n181 = To Fixed-Point(fixed-point type=w418, number=w420) -> (fixed-point=w419:fxp<+,32,-41>)
          n182 = Less Or Equal?(x=w419, y=w418) -> (x <= y?=w434:bool)
          n183 = Greater Or Equal?(x=w419, y=w435) -> (x >= y?=w433:bool)
          n184 = And(x=w434, y=w433) -> (x .and. y?=w432:bool)
          n185 = case shown="True" w432 {
            tunnel: [u8 7 ("Det 3") _] -> w431
            frame True {
            }
            frame False {
            }
          }
        }
        frame 7 {
          # "This section ensures that we only look for the particle\nwithin the speed bounds of the current filter"
          n186 = Increment(x=w443) -> (x+1=w442:T15)
          n187 = Unbundle By Name(w449) -> ("Gap Max Speed Count"=w447:i32)
          n188 = Unbundle By Name(w442) -> ("Detector Gap Count"=w448:i32)
          n189 = Greater Or Equal?(x=w448, y=w447) -> (x >= y?=w446:bool)
          n190 = case shown="True" w446 {
            tunnel: [u8 8 u8 7] -> w445
            frame True {
            }
            frame False {
            }
          }
        }
        frame 8 {
          # "Waits for a second detector correlation that's close to the\nfirst correlation, but make sure it's in the right speed range."
          n191 = Unbundle By Name(w456) -> ("First Correlation"=w459:i32)
          n192 = Increment(x=w457) -> (x+1=w454:T15)
          n193 = Unbundle By Name(w466) -> ("Gap Min Speed Count"=w465:i32)
          n194 = Unbundle By Name(w454) -> ("Detector Gap Count"=w458:i32)
          n195 = Add(x=w462, y=w461) -> (x+y=w455:i32)
          n196 = Greater?(x=w458, y=w465) -> (0:w464:bool)
          n197 = case shown="False" w464 {
            tunnel: [_ w477] -> w460
            tunnel: w463 -> [_ w476]
            tunnel: w452 -> [_ w473]
            tunnel: w459 -> [_ w468]
            frame True {
            }
            frame False {
              n198 = Unbundle By Name(w473) -> ("Det 2"=w467:i32)
              n199 = To Fixed-Point(number=w468) -> (fixed-point=w470:fxp<+/-,32,32>)  [unwired: 1 in]
              n200 = Subtract(x=fxp<+,1,1> 1.0, y=w476) -> (x-y=w474:fxp<+,12,2>)
              n201 = Multiply(x=w474, y=w470) -> (x*y=w472:fxp<+/-,43,33>)
              n202 = To Fixed-Point(number=w467) -> (fixed-point=w469:fxp<+/-,32,32>)  [unwired: 1 in]
              n203 = Greater?(x=w469, y=w472) -> (0:w471:bool)
              n204 = case shown="True" w471 {
                tunnel: [u8 9 u8 8] -> w477
                frame True {
                }
                frame False {
                }
              }
            }
          }
        }
        frame 9 {
          # "Waits for Boxcar 2 to reach the halfway point\nbetween Boxcars 1 and 3+4."
          n205 = Unbundle By Name(w505) -> ("Filter 1.Det 2"=w514:i32, "Filter 3.Det 2"=w517:i32, "Filter 4.Det 2"=w516:i32, "Filter 2.Det 2"=w508:i32)
          n206 = Increment(x=w490) -> (x+1=w485:T15)
          n207 = To Fixed-Point(number=w512) -> (fixed-point=w502:fxp<+/-,32,32>)  [unwired: 1 in]
          n208 = Unbundle By Name(w489) -> ("Gap Min Speed Count"=w487:i32)
          n209 = Unbundle By Name(w490) -> ("Detector Gap Count"=w488:i32)
          n210 = Decrement(x=w520) -> (x-1=w501:i32)
          n211 = Increment(x=w499) -> (x+1=w495:fxp<+,11,1>)
          n212 = Add(x=w517, y=w516) -> (x+y=w515:i32)
          n213 = Unbundle(w498) -> ("First Correlation"=w497:i32)  [unwired: 1 out]
          n214 = To Fixed-Point(number=w497) -> (fixed-point=w496:fxp<+/-,32,32>)  [unwired: 1 in]
          n215 = Add(x=w514, y=w515) -> (x+y=w518:i32)
          n216 = To Fixed-Point(number=w508) -> (fixed-point=w504:fxp<+/-,32,32>)  [unwired: 1 in]
          n217 = Unbundle By Name(w481) -> ("Det 2"=w480:i32)
          n218 = Multiply(x=w496, y=w495) -> (x*y=w493:fxp<+/-,43,33>)
          n219 = To Fixed-Point(number=w511) -> (fixed-point=w503:fxp<+/-,32,32>)  [unwired: 1 in]
          n220 = To Fixed-Point(number=w518) -> (fixed-point=w506:fxp<+/-,32,32>)  [unwired: 1 in]
          n221 = Multiply(x=w506, y=w502) -> (x*y=w513:fxp<+/-,64,64>)
          n222 = To Fixed-Point(number=w480) -> (fixed-point=w494:fxp<+/-,32,32>)  [unwired: 1 in]
          n223 = Scale By Power Of 2(n=i16 1, x=w503) -> (x*2^n=w509:fxp<+/-,32,32>)
          n224 = Greater Or Equal?(x=w488, y=w487) -> (x >= y?=w486:bool)
          n225 = Greater?(x=w494, y=w493) -> (0:w492:bool)
          n226 = Multiply(x=w504, y=w509) -> (x*y=w507:fxp<+/-,64,64>)
          n227 = Or(x=w492, y=w486) -> (x .or. y?=w491:bool)
          n228 = Greater?(x=w513, y=w507) -> (0:w500:bool)
          n229 = case shown="False" w500 {
            tunnel: [w525 u8 10 ("Det 3")] -> w519
            tunnel: w501 -> [w522 _]
            tunnel: w491 -> [w521 _]
            frame False {
              n230 = Less Or Equal To 0?(x=w522) -> (x <= 0?=w523:bool)
              n231 = Or(x=w521, y=w523) -> (x .or. y?=w524:bool)
              n232 = case shown="False" w524 {
                tunnel: [u8 9 ("Det 3") _] -> w525
                frame False {
                }
                frame True {
                }
              }
            }
            frame True {
            }
          }
          n233 = Bundle By Name(cluster=w485, "Second Detector Count"=0) -> (w484:T15)
        }
        frame 13 {
          # "Look carefully at the way the Armed variable is treated in here.\nIf One Shot implies Armed (ie, it's okay to let a particle through),\nthe particle is allowed to go through, but Armed is turned off."
          # "v = clockspeed * distance / speed count"
          # "1/2mv^2 = Vq\ntherefore\nm = 2Vq/v^2"
          n234 = Unbundle By Name(w529) -> ("First Detector Count"=w528:i32)
          n235 = Unbundle By Name(w557) -> ("High Velocity Limit"=w544:fxp<+,18,18>, "Low Velocity Limit"=w545:fxp<+,18,18>, "High Mass Limit"=w553:fxp<+,32,-37>, "Low Mass Limit"=w533:fxp<+,32,-37>, "High Voltage"=w548:fxp<+,22,22>)
          n236 = Multiply(x=w548, y=w535) -> (x*y=w554:fxp<+,54,-19>)
          n237 = To Fixed-Point(number=w528) -> (fixed-point=w543:fxp<+/-,32,32>)  [unwired: 1 in]
          n238 = To Fixed-Point(number=w528) -> (fixed-point=w536:fxp<+/-,32,32>)  [unwired: 1 in]
          n239 = Square(x=w536) -> (x^2=w537:fxp<+,63,63>)
          n240 = Multiply(x=w544, y=w543) -> (x*y=w542:fxp<+/-,50,50>)
          n241 = Multiply(x=w543, y=w545) -> (x*y=w541:fxp<+/-,50,50>)
          n242 = Multiply(x=w556, y=w537) -> (x*y=w555:fxp<+,64,19>)
          n243 = To Fixed-Point(fixed-point type=fxp<+,32,-13> 0.0, number=w555) -> (fixed-point=w531:fxp<+,32,-13>)
          n244 = Greater Or Equal?(x=w542, y=w534) -> (x >= y?=w552:bool)
          n245 = Less Or Equal?(x=w541, y=w534) -> (x <= y?=w551:bool)
          n246 = Multiply(x=w554, y=w531) -> (x*y=w538:fxp<+,64,-32>)
          n247 = Scale By Power Of 2(n=i16 1, x=w538) -> (x*2^n=w532:fxp<+,64,-32>)
          n248 = Less Or Equal?(x=w532, y=w553) -> (x <= y?=w550:bool)
          n249 = Greater Or Equal?(x=w532, y=w533) -> (x >= y?=w549:bool)
          n250 = Compound Arithmetic op=AND(w552, w551, w550, w549, w540) -> (w539:bool)
          n251 = case shown="True" w539 {
            tunnel: [u8 14 ("Det 3") _] -> w546
            frame True {
            }
            frame False {
            }
          }
        }
        frame 14 {
          # "I'm reusing outputs reduce LUT usage"
          # "To keep the names in the distance cluster from\ncorrupting the names of the speed counts cluster.\nThis really shouldn't happen, but it does."
          n252 = Unbundle By Name(w568) -> ("First Detector Count"=w574:i32)
          n253 = To Fixed-Point(number=w574) -> (fixed-point=w582:fxp<+/-,32,32>)  [unwired: 1 in]
          n254 = Multiply(x=w582, y=w581) -> (x*y=w580:T20)
          n255 = To Long Integer(number=w580) -> (32bit integer=w579:T21)
          n256 = Scale By Power Of 2(n=i16 -1, x=w572) -> (x*2^n=w573:i32)
          n257 = Subtract(x=w579, y=w578) -> (x-y=w577:T21)
          n258 = Subtract(x=w577, y=w573) -> (x-y=w570:T21)
          n259 = Unbundle By Name(w570) -> ("Distance to PSU"=w567:i32, "Distance to end of PSU"=w566:i32, "Distance to DCS 2"=w565:i32, "Distance to front of LEIL Chamber"=w561:i32, "Distance to DCS 1"=w559:i32)
          n260 = To Long Integer(number=w561) -> (32bit integer=w560:i32)
          n261 = To Long Integer(number=w567) -> (32bit integer=w564:i32)
          n262 = To Long Integer(number=w566) -> (32bit integer=w563:i32)
          n263 = To Long Integer(number=w565) -> (32bit integer=w562:i32)
          n264 = Add(x=w559, y=w575) -> ()  [unwired: 1 out]
          n265 = Bundle(cluster=w568, "First Detector Count"=w564, "Detector Gap Count"=w563, "Second Detector Count"=w562, "Second Detector Final Count"=w560) -> (w569:T15)
        }
        frame 15 {
          n266 = Decrement(x=w609) -> (x-1=w608:T15)
          n267 = Decrement(x=w591) -> (x-1=w584:i32)
          n268 = Unbundle(w608) -> ("First Detector Count"=w605:i32, "Detector Gap Count"=w603:i32, "Second Detector Count"=w600:i32, "Second Detector Final Count"=w598:i32)
          n269 = Add(x=w600, y=w588) -> (x+y=w601:i32)
          n270 = Add(x=w598, y=w588) -> (x+y=w587:i32)
          n271 = Add(x=w584, y=w588) -> (x+y=w586:i32)
          n272 = Less Or Equal To 0?(x=w600) -> (x <= 0?=w599:bool)
          n273 = Greater Or Equal To 0?(x=w587) -> (x >= 0?=w596:bool)
          n274 = Greater Or Equal To 0?(x=w586) -> (x >= 0?=w583:bool)
          n275 = Less Or Equal To 0?(x=w605) -> (x <= 0?=w604:bool)
          n276 = Less Or Equal To 0?(x=w598) -> (x <= 0?=w597:bool)
          n277 = Less Or Equal To 0?(x=w584) -> (x <= 0?=w585:bool)
          n278 = Greater Or Equal To 0?(x=w601) -> (x >= 0?=w593:bool)
          n279 = Greater Or Equal To 0?(x=w603) -> (x >= 0?=w602:bool)
          n280 = And(x=w597, y=w596) -> (x .and. y?=w590:bool)
          n281 = And(x=w585, y=w583) -> (x .and. y?=w589:bool)
          n282 = And(x=w604, y=w602) -> (x .and. y?=w607:bool)
          n283 = And(x=w599, y=w593) -> (x .and. y?=w606:bool)
          n284 = And(x=w592, y=w596) -> (x .and. y?=w594:bool)
          n285 = Compound Arithmetic op=OR(w594, w593, w583) -> (w595:bool)
          n286 = case shown="True" w595 {
            tunnel: [u8 15 ("Det 3") _] -> w610
            frame True {
            }
            frame False {
            }
          }
        }
      }
    }
    n287 = Delete From Array(array=w80) -> (array with subset deleted=w79:cluster{"Det 1":i16, "Det 2":i16}[])  [unwired: 2 in, 1 out]
    n288 = Or Array Elements(Boolean array=w122) -> (logical OR=w116:bool)
    n289 = Or Array Elements(Boolean array=w90) -> (logical OR=w96:bool)
    n290 = Or Array Elements(Boolean array=w125) -> (logical OR=w103:bool)
    n291 = Or Array Elements(Boolean array=w124) -> (logical OR=w100:bool)
    n292 = Or Array Elements(Boolean array=w123) -> (logical OR=w98:bool)
    n293 = Not(x=w116) -> (.not. x?=w121:bool)
    n294 = And(x=w121, y=w119) -> (x .and. y?=w120:bool)
    n295 = xnode ("Handshake Write")("Data"=w98, "Input Valid"=TRUE) -> ()  [unwired: 1 in, 2 out]
    n296 = xnode ("Handshake Write")("Data"=w103, "Input Valid"=TRUE) -> ()  [unwired: 1 in, 2 out]
    n297 = local write "Armed"(w120) -> ()
    n298 = Select(t=w75, s="Calibrate", f=w76) -> (s? t:f=w74:i32[])
    n299 = xnode ("Handshake Write")("Data"=w100, "Input Valid"=TRUE) -> ()  [unwired: 1 in, 2 out]
    n300 = xnode ("Handshake Write")("Data"=w96, "Input Valid"=TRUE) -> ()  [unwired: 1 in, 2 out]
  }
  n301 = node-c288(w42) -> ()
  n302 = node-c288(w28) -> ()
